vi "numeric.vi"(11 "input":dbl=1.1 caption="x") -> (3 "output":dbl)   [LabVIEW 2020]
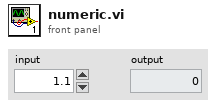
[diagram p1: front panel]
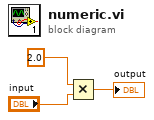
[diagram p0: block diagram]
diagram:
  n1 = Multiply(x=2.0, y="input") -> (x*y=→"output":dbl)
